vi "Move WindowTopLeft to MousePointer location.vi"(8 "error in (no error)":errorcluster) -> (0 "error out":errorcluster)   [LabVIEW 2012]
uses:
  <vilib>/Utility/inputDevices.llb/mouseAcquire.vi
  <vilib>/Utility/inputDevices.llb/closeMouse.vi
  <userlib>/_MGI/Application Control/MGI VI Reference/MGI Caller's VI Reference.vi
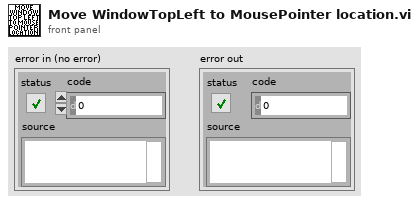
[diagram p1: front panel]
types:
  T1 = cluster{"Horizontal":i32, "Vertical":i32, "Scrolling":i32}
  T2 = typedef "LVRectTypeDef.ctl" = cluster{"Left":i16, "Top":i16, "Right":i16, "Bottom":i16}
  T3 = cluster{"Horizontal":i16, "Vertical":i16, "Scrolling":i16}
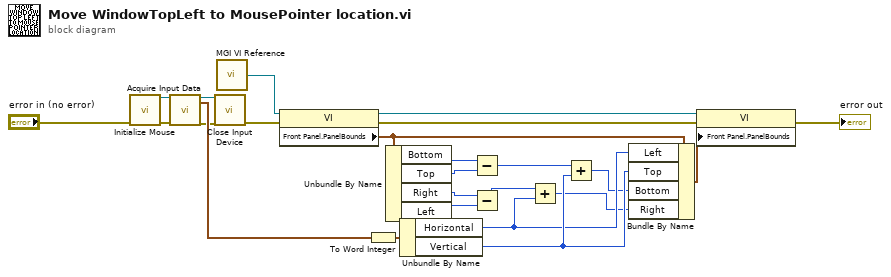
[diagram p0: block diagram]
diagram:
  n1 = call <vilib>:"Initialize Mouse.vi"("error in (no error)"="error in (no error)") -> ("error out"=w1:errorcluster, "device ID"=w2:refnum<k1>)  [unwired: 9 in]
  n2 = call-poly <vilib>:"Acquire Input Data.vi"("device ID"=w2, "error in (no error)"=w1) -> ("device ID"=w4:refnum<k1>, "axis info"=w5:T1, "error out"=w3:errorcluster)  [unwired: 14 in, 1 out]
  n3 = call-poly <vilib>:"Close Input Device.vi"("error in (no error)"=w3, "device ID"=w4) -> ("error out"=w16:errorcluster)  [unwired: 8 in]
  n4 = call-poly <userlib>:"MGI VI Reference.vi"() -> ("Caller's VI Reference"=w24:refnum<vi>)  [unwired: 1 in]
  n5 = property class="VI"(reference=w24, error in=w16) -> (reference out=w23:refnum<vi>, error out=w15:errorcluster, "Front Panel.PanelBounds"=w7:T2)
  n6 = To Word Integer(number=w5) -> (16bit integer=w12:T3)
  n7 = Unbundle By Name(w7) -> ("Bottom"=w8:i16, "Top"=w9:i16, "Right"=w10:i16, "Left"=w11:i16)
  n8 = Unbundle By Name(w12) -> ("Horizontal"=w19:i16, "Vertical"=w20:i16)
  n9 = Subtract(x=w8, y=w9) -> (x-y=w17:i16)
  n10 = Subtract(x=w10, y=w11) -> (x-y=w18:i16)
  n11 = Add(x=w18, y=w19) -> (x+y=w14:i16)
  n12 = Add(x=w17, y=w20) -> (x+y=w13:i16)
  n13 = Bundle By Name(cluster=w7, "Left"=w19, "Top"=w20, "Bottom"=w13, "Right"=w14) -> (w6:T2)
  n14 = property class="VI"(reference=w23, error in=w15, "Front Panel.PanelBounds"=w6) -> (error out=→"error out":errorcluster)  [unwired: 1 out]
